vi "GetImageType.vi"(8 "error in (no error)":errorcluster, 11 "CameraTestingProxyAPI in":refnum<class "CameraTestingProxyAPI.lvclass">) -> (0 "error out":errorcluster, 2 "ImageType":T1, 3 "CameraTestingProxyAPI out":refnum<class "CameraTestingProxyAPI.lvclass">)   [LabVIEW 2020, in "CameraTestingProxy.lvlib" / "CameraTestingProxyAPI.lvclass"]
uses:
  CameraTestingProxyAPI.lvclass
  ICameraTestingProxy/TypeDef/ImageType.ctl
  ICameraTestingProxy/TypeDef/Color Model.ctl
  CameraTestingProxyAPI.lvclass/CameraTestingProxyAPI.ctl
  9e12ebcf-0252-4f95-bf87-7d6c56462c03.vi
  ICameraTestingProxy/TypeDef/ICameraTestingProxy_typedef.lvlib
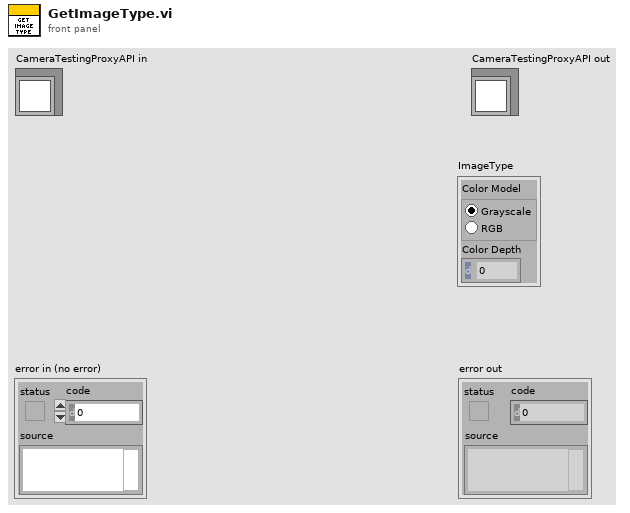
[diagram p1: front panel]
types:
  T1 = typedef "ICameraTestingProxy_typedef.lvlib/ImageType.ctl" = cluster{"Color Model":T2, "Color Depth":u8}
  T2 = typedef "ICameraTestingProxy_typedef.lvlib/Color Model.ctl" = enum32{"Greyscale", "RGB"}
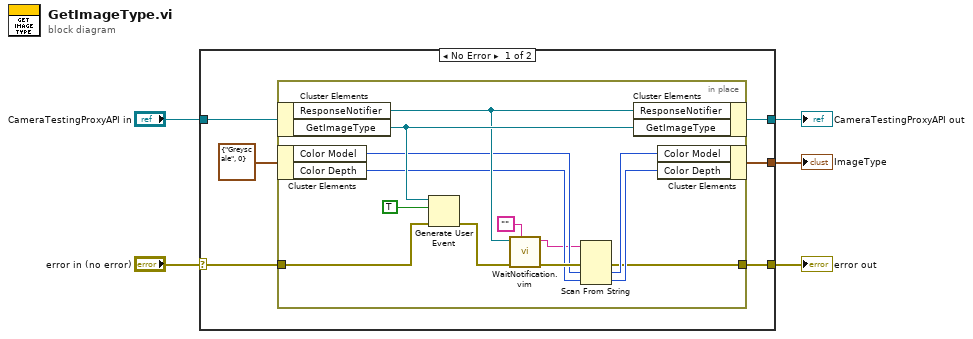
[diagram p0: block diagram]
diagram:
  n1 = case shown="No Error" "error in (no error)" {
    selector: "error in (no error)" -> [w9 w26]
    tunnel: "CameraTestingProxyAPI in" -> [w11 w25]
    tunnel: [w7 w26] -> w2
    tunnel: [w10 w25] -> w4
    tunnel: [w6 _] -> w1
    frame No Error {
      n2 = in-place {
        in-place-border: w9 -> [w24]
        in-place-border: [w14] -> w7
        n3 = in-place-cluster #1(w11) -> ("ResponseNotifier"=w20:refnum<notifier>, "GetImageType"=w21:refnum<user-event>)
        n4 = in-place-cluster #2(T1 {"Color Model"=enum."Greyscale", "Color Depth"=0} ("ImageType")) -> ("Color Model"=w18:T2, "Color Depth"=w17:u8)
        n5 = Generate User Event(user event=w21, event data cluster=TRUE ("event data"), error in=w24) -> (error out=w23:errorcluster)  [unwired: 1 in, 1 out]
        n6 = call "WaitNotification.vim"("Type"="", "error in (no error)"=w23, "ResponseNotifier"=w20) -> ("error out"=w19:errorcluster, "Data"=w12:string)  [unwired: 6 in, 1 out]
        n7 = Scan From String(input string=w12, error in=w19, default 1=w18, default 2=w17) -> (error out=w14:errorcluster, output 1=w16:T2, output 2=w15:u8)  [unwired: 2 in, 2 out]
        n8 = in-place-cluster #1("ResponseNotifier"=w20, "GetImageType"=w21) -> (w10:refnum<class "CameraTestingProxyAPI.lvclass">)
        n9 = in-place-cluster #2("Color Model"=w16, "Color Depth"=w15) -> (w6:T1)
      }
    }
    frame Error {
    }
  }
  "error out" <- w2
  "CameraTestingProxyAPI out" <- w4
  "ImageType" <- w1
